vi "UI_AutoRefresh_Init.vi"(8 "error in (no error)":errorcluster, 10 "Parameters":T1={"Write TipStrips with details (T)"=TRUE, "Write Captions with UserLabels (T)"=TRUE, "Mode (ind only)"=enum."Indicators only", "Enable nested stream (T)"=TRUE}, 11 "LiveDatActor in":refnum<class "LiveDatActor.lvclass">) -> (0 "error out":errorcluster, 3 "LiveDatActor out":refnum<class "LiveDatActor.lvclass">)   [LabVIEW 2020, in "LiveDatActor.lvlib" / "LiveDatActor.lvclass"]
uses:
  LiveDatActor.lvclass
  support/UI_Actor.lvlibp/UI_Actor/ctl_AR_Parameters.ctl
  support/UI_Actor.lvlibp/UI_Actor/ctl_AR_Mode.ctl
  LiveDatActor.lvclass/LiveDatActor.ctl
  support/Databox.lvlibp/TypesTools/Config/Read System Label.vi
  support/Databox.lvlibp/TypesTools/Config/Read User Label.vi
  support/Databox.lvlibp/TypesTools/Config/Read Unit.vi
  support/UI_Actor.lvlibp/UI_Actor/UI_Actor.lvclass
  support/Databox.lvlibp/TypesTools/Config/Config.lvclass
  D:/Projets/STEP AT/Bahamut/support/UI_Actor.lvlibp/UI_Actor/UI_Actor.lvclass
  D:/Projets/STEP AT/Bahamut/support/Actor Framework.lvlibp/1abvi3w/vi.lib/ActorFramework/Actor/Actor.lvclass
  D:/Projets/STEP AT/Bahamut/D&Cs/LiveDatActor/LiveDatActor/LiveDatActor.lvclass
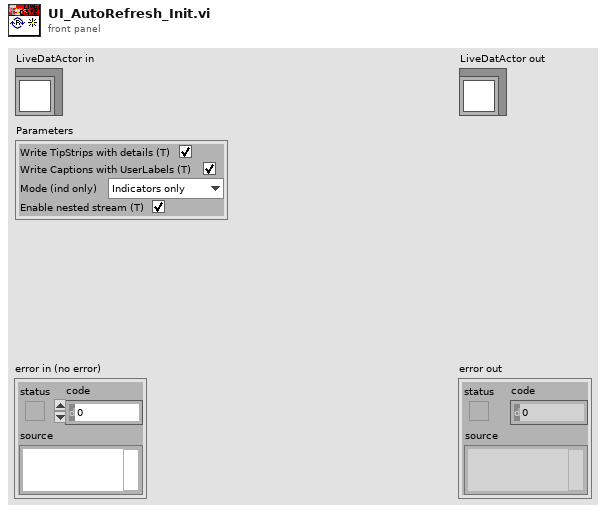
[diagram p1: front panel]
types:
  T1 = typedef "UI_Actor.lvlibp/UI_Actor.lvclass/ctl_AR_Parameters.ctl" = cluster{"Write TipStrips with details (T)":bool, "Write Captions with UserLabels (T)":bool, "Mode (ind only)":T2, "Enable nested stream (T)":bool}
  T2 = typedef "UI_Actor.lvlibp/UI_Actor.lvclass/ctl_AR_Mode.ctl" = enum16{"Controls only", "Indicators only", "All"}
  T3 = typedef "UI_Actor.lvlibp/UI_Actor.lvclass/ctl_InternalMapItem.ctl" = cluster{"Config":refnum<class "Config.lvclass">, "LatestData":refnum<class "Data.lvclass">}
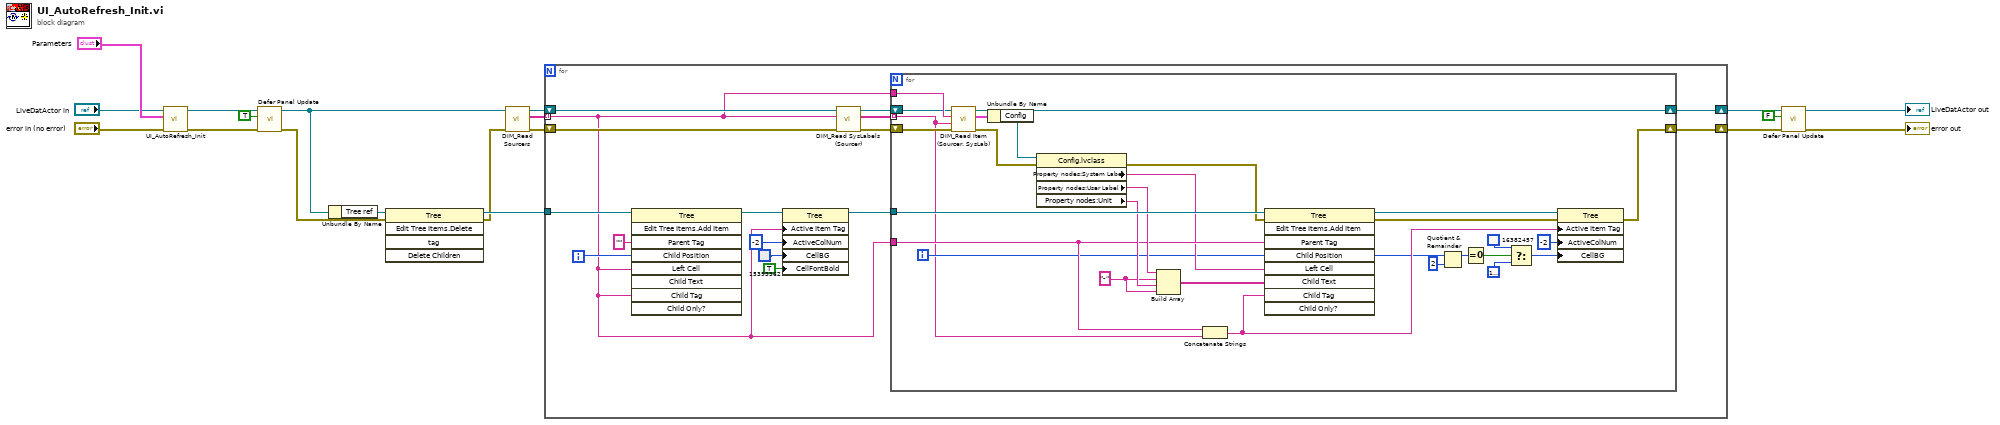
[diagram p0: block diagram]
diagram:
  n1 = call-parent "UI_AutoRefresh_Init.vi"("error in (no error)"="error in (no error)", "Parameters"="Parameters", "UI_Actor in"="LiveDatActor in") -> ("error out"=w3:errorcluster, "UI_Actor out"=w4:refnum<class "LiveDatActor.lvclass">)  [unwired: 7 in]
  n2 = call "Defer Panel Update.vi"("error in (no error)"=w3, "Defer Panel Updates"=TRUE, "UI_Actor in"=w4) -> ("error out"=w12:errorcluster, "UI_Actor out"=w11:refnum<class "LiveDatActor.lvclass">)  [unwired: 7 in]
  n3 = Unbundle By Name(w11) -> ("Tree ref"=w18:refnum<vi>)
  n4 = invoke class="Tree" method="Edit Tree Items.Delete"(reference=w18, error in=w12) -> (reference out=w17:refnum<vi>, error out=w14:errorcluster)  [unwired: 3 in, 3 out]
  n5 = call "DIM_Read Sourcers.vi"("error in (no error)"=w14, "UI_Actor in"=w11) -> ("error out"=w13:errorcluster, "DIM Sourcers"=w16:string[], "UI_Actor out"=w15:refnum<class "LiveDatActor.lvclass">)  [unwired: 7 in]
  n6 = for {
    tunnel: w17 -> [w35]
    tunnel: w16 -> [w21] mode=indexing
    shift-right: [w26] -> w8
    shift-left: w15 -> [w32]
    shift-right: [w27] -> w7
    shift-left: w13 -> [w29]
    i -> [w33]
    n7 = invoke class="Tree" method="Edit Tree Items.Add Item"(reference=w35, "Parent Tag"="", "Child Position"=w33, "Left Cell"=w21, "Child Tag"=w21) -> (reference out=w24:refnum<vi>)  [unwired: 4 in, 8 out]
    n8 = property class="Tree"(reference=w24, "Active Item Tag"=w21, "ActiveColNum"=-2 ("Active Cell:Active Column Number"), "CellBG"=u32 15395562, "CellFontBold"=TRUE ("Active Cell:Cell Font:Bold")) -> (reference out=w23:refnum<vi>)  [unwired: 1 in, 1 out]
    n9 = call "DIM_Read SysLabels (Sourcer).vi"("error in (no error)"=w29, "Sourcer"=w21, "UI_Actor in"=w32) -> ("error out"=w28:errorcluster, "DIM Sourcer's SysLabels"=w31:string[], "UI_Actor out"=w30:refnum<class "LiveDatActor.lvclass">)  [unwired: 6 in]
    n10 = for {
      tunnel: w31 -> [w36] mode=indexing
      tunnel: w21 -> [w50]
      tunnel: w23 -> [w63]
      tunnel: w21 -> [w62]
      shift-right: [w56] -> w26
      shift-left: w30 -> [w61]
      shift-right: [w37] -> w27
      shift-left: w28 -> [w57]
      i -> [w46]
      w52 = "-"
      n11 = call "DIM_Read Item (Sourcer, SysLab).vi"("error in (no error)"=w57, "SysLabel"=w36, "Sourcer"=w62, "UI_Actor in"=w61) -> ("error out"=w54:errorcluster, "DIM Item"=w60:T3, "UI_Actor out"=w56:refnum<class "LiveDatActor.lvclass">)  [unwired: 4 in, 1 out]
      n12 = Unbundle By Name(w60) -> ("Config"=w59:refnum<class "Config.lvclass">)
      n13 = property class="Config.lvclass"(reference=w59, error in=w54) -> (error out=w55:errorcluster, "Property nodes:System Label"=w49:string, "Property nodes:User Label"=w51:string, "Property nodes:Unit"=w53:string)  [unwired: 1 out]
      n14 = Build Array(w51, w52, w53, w52) -> (w58:string[])
      n15 = Concatenate Strings(w50, w36) -> (w48:string)
      n16 = invoke class="Tree" method="Edit Tree Items.Add Item"(reference=w63, error in=w55, "Parent Tag"=w50, "Child Position"=w46, "Left Cell"=w49, "Child Text"=w58, "Child Tag"=w48) -> (reference out=w39:refnum<vi>, error out=w38:errorcluster)  [unwired: 2 in, 7 out]
      n17 = Quotient & Remainder(x=w46, y=2) -> (x-y*floor(x/y)=w44:i32)  [unwired: 1 out]
      n18 = Equal To 0?(x=w44) -> (x = 0?=w43:bool)
      n19 = Select(t=u32 16382457, s=w43, f=u32 16777226) -> (s? t:f=w40:u32)
      n20 = property class="Tree"(reference=w39, error in=w38, "Active Item Tag"=w48, "ActiveColNum"=-2 ("Active Cell:Active Column Number"), "CellBG"=w40) -> (error out=w37:errorcluster)  [unwired: 1 out]
    }
  }
  n21 = call "Defer Panel Update.vi"("error in (no error)"=w7, "Defer Panel Updates"=FALSE, "UI_Actor in"=w8) -> ("error out"=→"error out":errorcluster, "UI_Actor out"=→"LiveDatActor out":refnum<class "LiveDatActor.lvclass">)  [unwired: 7 in]
